vi "Resonant X-Stretch Compensation.vi"(7 "Excess X_Pixels (if ZOOM <1)":T1, 8 "Reso Phase correction factor":dbl, 9 "Start Delay (Ticks)":dbl, 10 "X Pixel Array IN":i16[](array[numeric]), 11 "Image Ref IN":T2) -> (2 "X-Stretched Array OUT":i16[](array[numeric]), 3 "Corrected Image Out":T2)   [LabVIEW 2012]
uses:
  <vilib>/vision/Image Controls.llb/IMAQ Image.ctl
  <vilib>/vision/NI_Vision_Development_Module.lvlib
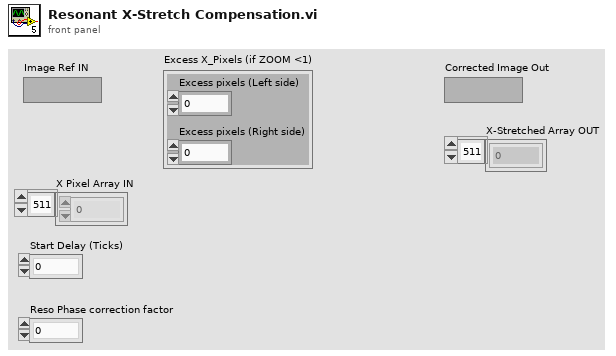
[diagram p1: front panel]
types:
  T1 = cluster{"Excess pixels (Left side)":i32, "Excess pixels (Right side)":i32}
  T2 = typedef "IMAQ Image.ctl" = refnum<image>
  T3 = typedef "Image Type" = u32
  T4 = cluster{"window size":i32, "resample size":i32}[]
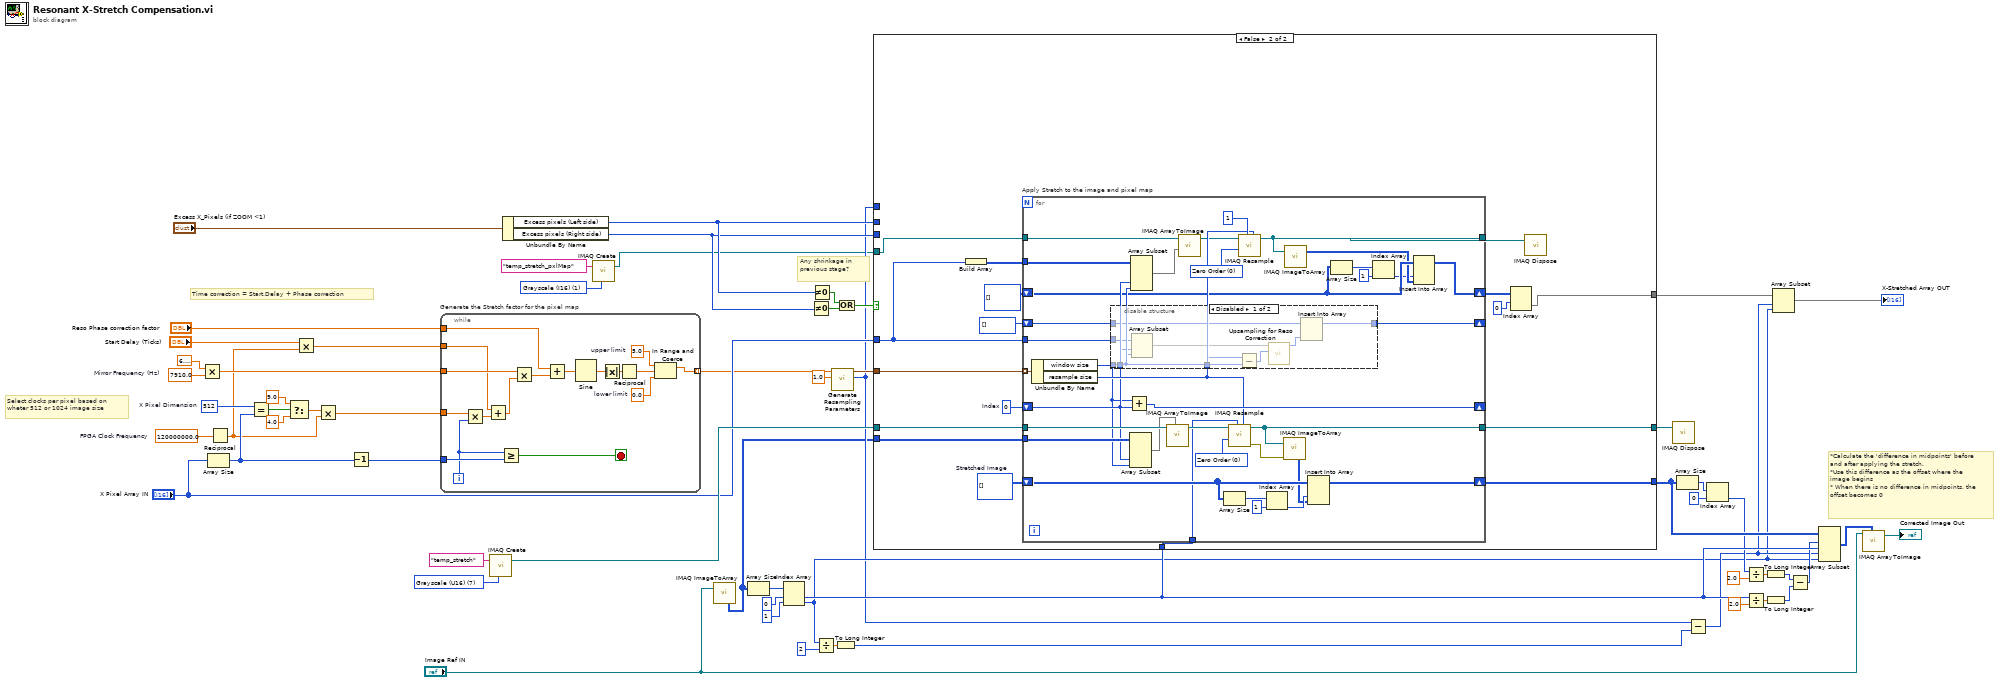
[diagram p0: block diagram]
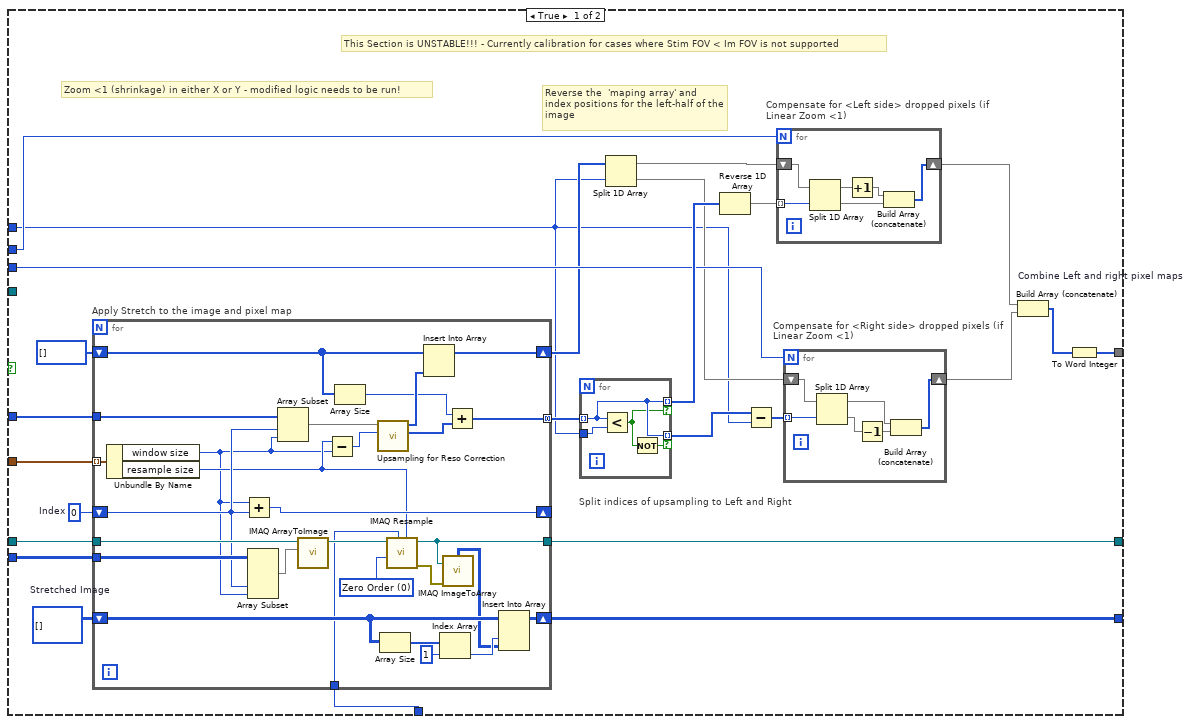
[diagram p2: hidden frame]
diagram:
  w5 = T3 1 items=["Grayscale (U8)", "Grayscale (I16)", "Grayscale (SGL)", "Complex (CSG)", "RGB (U32)", "HSL (U32)", "RGB (U64)", "Grayscale (U16)"] ("Image Type")
  w49 = T3 7 items=["Grayscale (U8)", "Grayscale (I16)", "Grayscale (SGL)", "Complex (CSG)", "RGB (U32)", "HSL (U32)", "RGB (U64)", "Grayscale (U16)"] ("Image Type")
  w41 = 512  # X Pixel Dimension
  w57 = 120000000.0  # FPGA Clock Frequency
  w58 = 7910.0  # Mirror Frequency (Hz)
  # "Any shrinkage in previous stage?"
  # "Time correction = Start.Delay + Phase correction"
  # "*Calculate the 'difference in midpoints' before and after applying the stretch.\n*Use this difference as the offset where the image begins\n* When there is no difference in midpoints, the offset becomes 0"
  # "Select clocks per pixel based on wheter 512 or 1024 image size"
  n1 = Multiply(x=6.283185307179586, y=w58) -> (x*y=w59:dbl)
  n2 = Array Size(array="X Pixel Array IN") -> (size(s)=w40:i32)
  n3 = Reciprocal(x=w57) -> (1/x=w21:dbl)
  n4 = Equal?(x=w41, y=w40) -> (x = y?=w55:bool)
  n5 = Select(t=9.0 ("clocks per pixel"), s=w55, f=4.0) -> (s? t:f=w39:dbl)
  n6 = Multiply(x="Start Delay (Ticks)", y=w21) -> (x*y=w19:dbl)
  n7 = Multiply(x=w39, y=w21) -> (x*y=w56:dbl)
  n8 = Decrement(x=w40) -> (x-1=w42:i32)
  n9 = while "Generate the Stretch factor for the pixel map" {
    tunnel: w56 -> [w77]
    tunnel: w59 -> [w76]
    tunnel: [w61] -> w7 mode=indexing
    tunnel: w42 -> [w73]
    tunnel: w19 -> [w69]
    tunnel: "Reso Phase correction factor" -> [w66]
    i -> [w71]
    stop <- w72 stop-if-true
    w62 = 5.0  # upper limit
    w63 = 0.0  # lower limit
    n10 = Multiply(x=w77, y=w71) -> (x*y=w70:dbl)
    n11 = Add(x=w69, y=w70) -> (x+y=w68:dbl)
    n12 = Greater Or Equal?(x=w71, y=w73) -> (x >= y?=w72:bool)
    n13 = Multiply(x=w76, y=w68) -> (x*y=w67:dbl)
    n14 = Add(x=w66, y=w67) -> (x+y=w65:dbl)
    n15 = Sine(x=w65) -> (sin(x)=w75:dbl)
    n16 = Absolute Value(x=w75) -> (abs(x)=w74:dbl)
    n17 = Reciprocal(x=w74) -> (1/x=w64:dbl)
    n18 = In Range and Coerce(upper limit=w62, x=w64, lower limit=w63) -> (coerced(x)=w61:dbl)  [unwired: 1 out]
  }
  n19 = call "IMAQ Create"("Image Name"="temp_stretch", "Image Type"=w49) -> ("New Image"=w35:T2)  [unwired: 3 in, 1 out]
  n20 = Unbundle By Name("Excess X_Pixels (if ZOOM <1)") -> ("Excess pixels (Left side)"=w9:i32, "Excess pixels (Right side)"=w8:i32)
  n21 = call "IMAQ Create"("Image Name"="temp_stretch_pxlMap", "Image Type"=w5) -> ("New Image"=w3:T2)  [unwired: 3 in, 1 out]
  n22 = call "IMAQ ImageToArray"("Image"="Image Ref IN") -> ("Image Pixels (U16)"=w2:u16[][])  [unwired: 3 in, 4 out]
  n23 = Array Size(array=w2) -> (size(s)=w52:i32[])
  n24 = Index Array(array=w52, index #1=0 ("index"), index #2=1 ("index")) -> (element #1=w34:i32, element #2=w14:i32)
  n25 = Not Equal To 0?(x=w8) -> (x != 0?=w11:bool)
  n26 = Not Equal To 0?(x=w9) -> (x != 0?=w12:bool)
  n27 = Divide(x=w14, y=2) -> (x/y=w44:dbl)
  n28 = call "Generate Resampling Parameters.vi"("X.ZOOM (Linear)"=1.0 ("X.ZOOM"), "Stretch Array IN"=w7) -> ("Modified Midpoint pixel (After stretch)"=w6:i32, "Window size and Resampling OUT"=w38:T4)  [unwired: 8 in]
  n29 = To Long Integer(number=w44) -> (32bit integer=w43:i32)
  n30 = Or(x=w12, y=w11) -> (x .or. y?=w10:bool)
  n31 = case shown="False" w10 {
    tunnel: [w102 w163] -> w46
    tunnel: w2 -> [w101 w162]
    tunnel: w38 -> [w100 w161]
    tunnel: [w97 w158] -> w37
    tunnel: w35 -> [w96 w157]
    tunnel: w34 -> [w95 w156]
    tunnel: "X Pixel Array IN" -> [w94 w147]
    tunnel: [w78 w148] -> w17
    tunnel: w9 -> [w92 _]
    tunnel: w8 -> [w87 _]
    tunnel: w6 -> [w83 _]
    tunnel: w3 -> [_ w153]
    frame True {
      w98 = u8[][] []  # Stretched Image
      w99 = 0  # Index
      # "This Section is UNSTABLE!!! - Currently calibration for cases where Stim FOV < Im FOV is not supported"
      # "Zoom <1 (shrinkage) in either X or Y - modified logic needs to be run!"
      # "Reverse the  'maping array' and  \nindex positions for the left-half of the image"
      n32 = for "Apply Stretch to the image and pixel map" {
        tunnel: w100 -> [w146] mode=indexing
        tunnel: w101 -> [w145]
        shift-right: [w144] -> _
        shift-left: w99 -> [w129]
        shift-right: [w143] -> w102
        shift-left: w98 -> [w142]
        tunnel: w96 -> [w135]
        tunnel: w95 -> [w132]
        tunnel: [w131] -> w97
        shift-right: [w123] -> w86
        shift-left: i32[] [] ("X Pixel Array IN") -> [w122]
        tunnel: w94 -> [w130]
        tunnel: [w119] -> w91 mode=concatenating
        w138 = u32 0 items=["Zero Order", "Bi-Linear", "Quadratic", "Cubic Spline"] ("Interpolation Type")
        n33 = Unbundle By Name(w146) -> ("window size"=w126:i32, "resample size"=w127:i32)
        n34 = Add(x=w126, y=w129) -> (x+y=w144:i32)
        n35 = Array Subset(array=w145, index (col)=w129, length (col)=w126) -> (w136:u16[][])  [unwired: 2 in]
        n36 = Array Subset(array=w130, index=w129, length=w126) -> (w128:i16[])
        n37 = call "IMAQ ArrayToImage"("Image Pixels (U8)"=w136, "Image"=w135) -> ("Image Out"=w134:T2)  [unwired: 8 in, 1 out]
        n38 = Subtract(x=w127, y=w126) -> (x-y=w125:i32)
        n39 = Array Size(array=w122) -> (size(s)=w121:i32)
        n40 = call "Upsampling for Reso Correction.vi"("Extra points"=w125, "Pixel Map IN"=w128) -> ("Insert Positions OUT"=w120:i32[], "Pixel Map OUT (Zoomed in)"=w124:i32[])  [unwired: 8 in]
        n41 = Array Size(array=w142) -> (size(s)=w141:i32[])
        n42 = call "IMAQ Resample"("X Resolution"=w127, "Y Resolution"=w132, "Interpolation Type"=w138, "Image Src"=w134) -> ("error out"=w137:errorcluster, "Image Dst Out"=w131:T2)  [unwired: 6 in]
        n43 = Insert Into Array(array=w122, new element=w124) -> (w123:i32[])  [unwired: 1 in]
        n44 = Index Array(array=w141, index=1) -> (element=w139:i32)
        n45 = call "IMAQ ImageToArray"("error in (no error)"=w137, "Image"=w131) -> ("Image Pixels (U8)"=w133:u8[][])  [unwired: 2 in, 4 out]
        n46 = Add(x=w121, y=w120) -> (x+y=w119:i32[])
        n47 = Insert Into Array(array=w142, index (col)=w139, new element=w133) -> (w143:u8[][])  [unwired: 1 in]
      }
      n48 = for "Split indices of upsampling to Left and Right" {
        tunnel: w91 -> [w111] mode=indexing
        tunnel: w83 -> [w112]
        tunnel: [w111] -> w90 mode=indexing if=w109
        tunnel: [w111] -> w84 mode=indexing if=w110
        n49 = Less?(x=w111, y=w112) -> (x < y?=w109:bool)
        n50 = Not(x=w109) -> (.not. x?=w110:bool)
      }
      n51 = Split 1D Array(array=w86, index=w83) -> (first subarray=w81:i32[], second subarray=w85:i32[])
      n52 = Reverse 1D Array(array=w90) -> (reversed array=w89:i32[])
      n53 = Subtract(x=w84, y=w83) -> (x-y=w82:i32[])
      n54 = for "Compensate for <Left side> dropped pixels (if Linear Zoom <1)" {
        N: w92 -> [_]
        tunnel: w89 -> [w117] mode=indexing
        shift-right: [w116] -> w80
        shift-left: w81 -> [w118]
        n55 = Split 1D Array(array=w118, index=w117) -> (first subarray=w114:i32[], second subarray=w115:i32[])
        n56 = Increment(x=w114) -> (x+1=w113:i32[])
        n57 = Build Array (concatenate)(w113, w115) -> (w116:i32[])
      }
      n58 = for "Compensate for <Right side> dropped pixels (if Linear Zoom <1)" {
        N: w87 -> [_]
        shift-right: [w104] -> w88
        shift-left: w85 -> [w108]
        tunnel: w82 -> [w103] mode=indexing
        n59 = Split 1D Array(array=w108, index=w103) -> (first subarray=w105:i32[], second subarray=w107:i32[])
        n60 = Decrement(x=w107) -> (x-1=w106:i32[])
        n61 = Build Array (concatenate)(w105, w106) -> (w104:i32[])
      }
      n62 = Build Array (concatenate) "Combine Left and right pixel maps"(w80, w88) -> (w79:i32[])
      n63 = To Word Integer(number=w79) -> (16bit integer=w78:i16[])
    }
    frame False {
      w159 = u16[][] []  # Stretched Image
      w160 = 0  # Index
      n64 = Build Array(w147) -> (w151:i16[][])
      n65 = for "Apply Stretch to the image and pixel map" {
        tunnel: w161 -> [w198] mode=indexing
        tunnel: w162 -> [w197]
        shift-right: [w196] -> _
        shift-left: w160 -> [w175]
        shift-right: [w195] -> w163
        shift-left: w159 -> [w194]
        tunnel: w157 -> [w188]
        tunnel: w156 -> [w186]
        tunnel: [w185] -> w158
        shift-right: [w182] -> _
        shift-left: i32[] [] ("X Pixel Array IN") -> [w183]
        tunnel: w147 -> [w184]
        shift-right: [w168] -> w150
        shift-left: i16[][] [] ("X Pixel Array IN") -> [w169]
        tunnel: w153 -> [w178]
        tunnel: [w172] -> w152
        tunnel: w151 -> [w176]
        w179 = u32 0 items=["Zero Order", "Bi-Linear", "Quadratic", "Cubic Spline"] ("Interpolation Type")
        w190 = u32 0 items=["Zero Order", "Bi-Linear", "Quadratic", "Cubic Spline"] ("Interpolation Type")
        n66 = Unbundle By Name(w198) -> ("window size"=w174:i32, "resample size"=w180:i32)
        n67 = disable-structure shown="Disabled" {
          disable-tunnel: w184 -> [w207 _]
          disable-tunnel: w183 -> [w204 w208]
          disable-tunnel: [w202 w208] -> w182
          disable-tunnel: w180 -> [w201 _]
          disable-tunnel: w175 -> [w200 _]
          disable-tunnel: w174 -> [w199 _]
          frame Disabled {
            n68 = Array Subset(array=w207, index=w200, length=w199) -> (w206:i16[])
            n69 = Subtract(x=w201, y=w199) -> (x-y=w205:i32)
            n70 = call "Upsampling for Reso Correction.vi"("Extra points"=w205, "Pixel Map IN"=w206) -> ("Pixel Map OUT (Zoomed in)"=w203:i32[])  [unwired: 8 in, 1 out]
            n71 = Insert Into Array(array=w204, new element=w203) -> (w202:i32[])  [unwired: 1 in]
          }
          frame Enabled {
          }
        }
        n72 = Add(x=w174, y=w175) -> (x+y=w196:i32)
        n73 = Array Subset(array=w197, index (col)=w175, length (col)=w174) -> (w164:u16[][])  [unwired: 2 in]
        n74 = Array Subset(array=w176, index (col)=w175, length (col)=w174) -> (w173:i16[][])  [unwired: 2 in]
        n75 = call "IMAQ ArrayToImage"("Image Pixels (U16)"=w164, "Image"=w188) -> ("Image Out"=w187:T2)  [unwired: 8 in, 1 out]
        n76 = call "IMAQ ArrayToImage"("Image Pixels (I16)"=w173, "Image"=w178) -> ("Image Out"=w177:T2)  [unwired: 8 in, 1 out]
        n77 = Array Size(array=w194) -> (size(s)=w193:i32[])
        n78 = call "IMAQ Resample"("X Resolution"=w180, "Y Resolution"=w186, "Interpolation Type"=w190, "Image Src"=w187) -> ("error out"=w189:errorcluster, "Image Dst Out"=w185:T2)  [unwired: 6 in]
        n79 = call "IMAQ Resample"("X Resolution"=w180, "Y Resolution"=1, "Interpolation Type"=w179, "Image Src"=w177) -> ("Image Dst Out"=w172:T2)  [unwired: 6 in, 1 out]
        n80 = Index Array(array=w193, index=1) -> (element=w191:i32)
        n81 = call "IMAQ ImageToArray"("error in (no error)"=w189, "Image"=w185) -> ("Image Pixels (U16)"=w165:u16[][])  [unwired: 2 in, 4 out]
        n82 = call "IMAQ ImageToArray"("Image"=w172) -> ("Image Pixels (I16)"=w167:i16[][])  [unwired: 3 in, 4 out]
        n83 = Insert Into Array(array=w194, index (col)=w191, new element=w165) -> (w195:u16[][])  [unwired: 1 in]
        n84 = Array Size(array=w169) -> (size(s)=w170:i32[])
        n85 = Index Array(array=w170, index=1) -> (element=w166:i32)
        n86 = Insert Into Array(array=w169, index (col)=w166, new element=w167) -> (w168:i16[][])  [unwired: 1 in]
      }
      n87 = Index Array(array=w150, index (row)=0 ("index")) -> (element=w148:i16[])  [unwired: 1 in]
      n88 = call "IMAQ Dispose"("Image"=w152) -> ()  [unwired: 5 in, 1 out]
    }
  }
  n89 = call "IMAQ Dispose"("Image"=w37) -> ()  [unwired: 5 in, 1 out]
  n90 = Array Size(array=w46) -> (size(s)=w32:i32[])
  n91 = Subtract(x=w6, y=w43) -> (x-y=w15:i32)
  n92 = Index Array(array=w32, index=0) -> (element=w30:i32)
  n93 = Divide(x=w30, y=2.0) -> (x/y=w28:dbl)
  n94 = Divide(x=w34, y=2.0) -> (x/y=w27:dbl)
  n95 = To Long Integer(number=w28) -> (32bit integer=w25:i32)
  n96 = To Long Integer(number=w27) -> (32bit integer=w24:i32)
  n97 = Array Subset(array=w17, index=w15, length=w14) -> (→"X-Stretched Array OUT":i16[])
  n98 = Subtract(x=w25, y=w24) -> (x-y=w23:i32)
  n99 = Array Subset(array=w46, index (row)=w23, length (row)=w34, index (col)=w15, length (col)=w14) -> (w1:u16[][])
  n100 = call "IMAQ ArrayToImage"("Image Pixels (U16)"=w1, "Image"="Image Ref IN") -> ("Image Out"=→"Corrected Image Out":T2)  [unwired: 8 in, 1 out]
